vi "PushValves.vi"(6 "StartTime":timestamp, 8 "Valves":refnum<vi>, 11 "Array":string[](array[string])) -> (0 "Current Time":dbl, 3 "Enqueue":string)   [LabVIEW 2019, in "Scripts.lvclass"]
uses:
  Scripts.lvclass
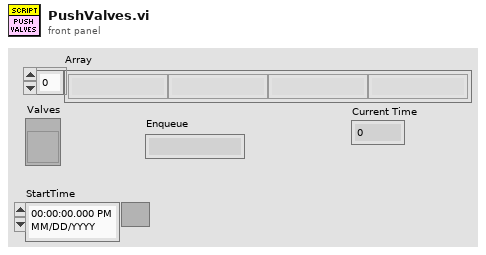
[diagram p1: front panel]
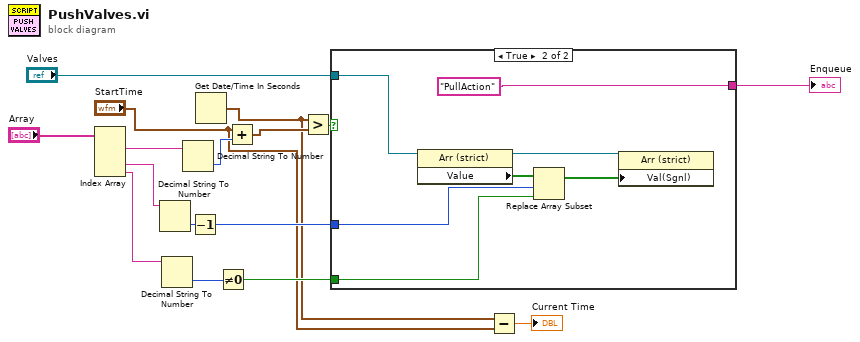
[diagram p0: block diagram]
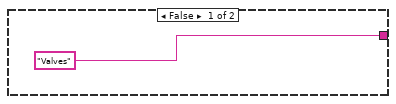
[diagram p2: hidden frame]
diagram:
  n1 = Index Array(array="Array") -> (element #1=w15:string, element #3=w8:string, element #4=w11:string)  [unwired: 4 in, 1 out]
  n2 = Decimal String To Number(string=w8) -> (number=w7:i32)  [unwired: 2 in, 1 out]
  n3 = Decimal String To Number(string=w11) -> (number=w10:i32)  [unwired: 2 in, 1 out]
  n4 = Decimal String To Number(string=w15) -> (number=w14:i32)  [unwired: 2 in, 1 out]
  n5 = Decrement(x=w7) -> (x-1=w6:i32)
  n6 = Get Date/Time In Seconds() -> (seconds since 1Jan1904=w2:timestamp)
  n7 = Not Equal To 0?(x=w10) -> (x != 0?=w9:bool)
  n8 = Add(x="StartTime", y=w14) -> (x+y=w4:timestamp)
  n9 = Greater?(x=w2, y=w4) -> (0:w13:bool)
  n10 = case shown="True" w13 {
    tunnel: ["Valves" ("element") "PullAction" ("element")] -> w12
    tunnel: w9 -> [_ w20]
    tunnel: w6 -> [_ w21]
    tunnel: "Valves" -> [_ w23]
    frame False {
    }
    frame True {
      n11 = property class="Arr (strict)"(reference=w23) -> (reference out=w18:refnum<vi>, "Value"=w22:bool[])  [unwired: 1 in, 1 out]
      n12 = Replace Array Subset(array=w22, new element=w20, index=w21) -> (w19:bool[])
      n13 = property class="Arr (strict)"(reference=w18, "Val(Sgnl)"=w19) -> ()  [unwired: 1 in, 2 out]
    }
  }
  "Enqueue" <- w12
  n14 = Subtract(x=w2, y="StartTime") -> (x-y=→"Current Time":dbl)
